vi "Convert Alarm Cluster.vi"(11 "alarm data in":T2(array[cluster]) {"value" format="%.2f"; "setpoint" format="%.2f"; "clear time" format="%<%X\n%x>T"; "ack time" format="%<%X\n%x>T"; "set time" format="%<%X\n%x>T"}) -> (3 "alarms out":T1(array[cluster]) {"value" format="%.2f"; "setpoint" format="%.2f"; "clear time" format="%<%X\n%x>T"; "ack time" format="%<%X\n%x>T"; "set time" format="%<%X\n%x>T"})   [LabVIEW 2018, in "Dynamic Shared Variables.lvlib"]
doc: "NI goofed and used two different cluster orders for Alarm & Event Query.vi and Read Alarms.vi.\nThis VI converts from one to the other."
uses:
  Dynamic Shared Variables.lvlib
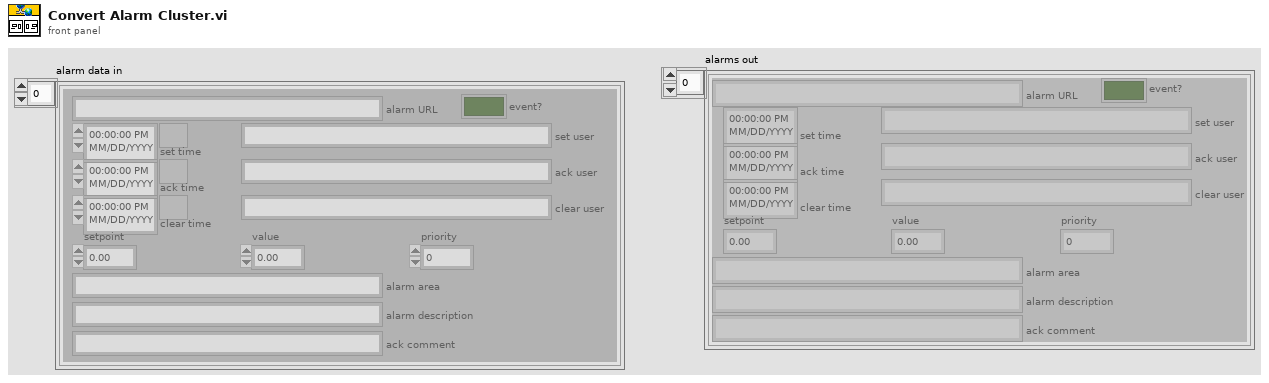
[diagram p1: front panel]
types:
  T1 = cluster{"alarm URL":string, "set time":timestamp, "set user":string, "ack time":timestamp, "ack user":string, "clear time":timestamp, "clear user":string, "setpoint":dbl, "value":dbl, "priority":u32, "alarm area":string, "alarm description":string, "ack comment":string, "event?":bool, "Refnum":u64}[]
  T2 = cluster{"alarm URL":string, "set time":timestamp, "set user":string, "ack time":timestamp, "ack user":string, "clear time":timestamp, "clear user":string, "setpoint":dbl, "value":dbl, "priority":u32, "alarm area":string, "alarm description":string, "ack comment":string, "Refnum":u32, "event?":bool}[]
  T3 = cluster{"alarm URL":string, "set time":timestamp, "set user":string, "ack time":timestamp, "ack user":string, "clear time":timestamp, "clear user":string, "setpoint":dbl, "value":dbl, "priority":u32, "alarm area":string, "alarm description":string, "ack comment":string, "event?":bool, "Refnum":u64}
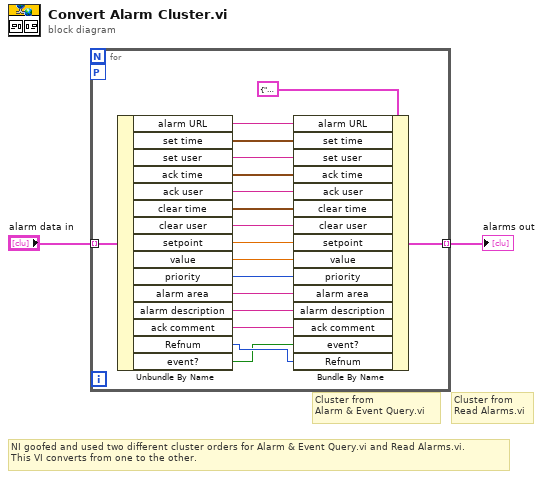
[diagram p0: block diagram]
diagram:
  # "NI goofed and used two different cluster orders for Alarm & Event Query.vi and Read Alarms.vi.\nThis VI converts from one to the other."
  # "Cluster from \nRead Alarms.vi"
  # "Cluster from\nAlarm & Event Query.vi"
  n1 = for {
    tunnel: "alarm data in" -> [w20] mode=indexing
    tunnel: [w17] -> w1 mode=indexing
    workers-P: _ -> [_]
    n2 = Unbundle By Name(w20) -> ("alarm URL"=w18:string, "set time"=w16:timestamp, "set user"=w15:string, "ack time"=w14:timestamp, "ack user"=w13:string, "clear time"=w12:timestamp, "clear user"=w11:string, "setpoint"=w10:dbl, "value"=w9:dbl, "priority"=w8:u32, "alarm area"=w7:string, "alarm description"=w6:string, "ack comment"=w5:string, "Refnum"=w4:u32, "event?"=w3:bool)
    n3 = Bundle By Name(cluster=T3 {"alarm URL"="", "set time"=timestamp(0 s since 1904-01-01), "set user"="", "ack time"=timestamp(0 s since 1904-01-01), "ack user"="", "clear time"=timestamp(0 s since 1904-01-01), "clear user"="", "setpoint"=0.0, "value"=0.0, "priority"=0, "alarm area"="", "alarm description"="", "ack comment"="", "event?"=FALSE, "Refnum"=0} ("Alarm"), "alarm URL"=w18, "set time"=w16, "set user"=w15, "ack time"=w14, "ack user"=w13, "clear time"=w12, "clear user"=w11, "setpoint"=w10, "value"=w9, "priority"=w8, "alarm area"=w7, "alarm description"=w6, "ack comment"=w5, "event?"=w3, "Refnum"=w4) -> (w17:T3)
  }
  "alarms out" <- w1
